vi "T7_WriteRead_FLOAT32_Test_Register.vi"() -> ()   [LabVIEW 2014]
uses:
  Serial Link Layer/NI_Modbus_Cleaned/NI Modbus121Clean.llb/MB Ethernet Master Query Read Input Registers (poly).vi
  Serial Link Layer/NI_Modbus_Cleaned/NI Modbus121Clean.llb/MB Ethernet Master Query Write Multiple Registers (poly).vi
panel:
  in  "LabJack TestFLOAT32 Register":i32=55124
  out "Read FLOAT32":sgl
  out "Raw Data Read":u16[](array[numeric])
  in  "FLOAT32 to Write":sgl=1.23
  in  "WriteData":bool
  in  "Remote IP Address":string="192.168.1.15"
  in  "Remote Port":u16=502
  in  "Stop":bool
  # "MB Ethernet Example Master.vi\n\nInstructions\n1.Use Kipling to find your devices IP address & modify the\n\"Remote IP Addres\"\n2. Run this VI\n3. Change value of \"FLOAT32 to Write\" & press \"Write Data\""
  # "TCP Parameters"
  # "Test Write & Read of TEST_UINT32 Register"
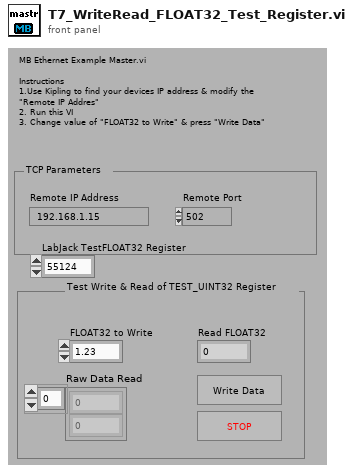
[diagram p1: front panel]
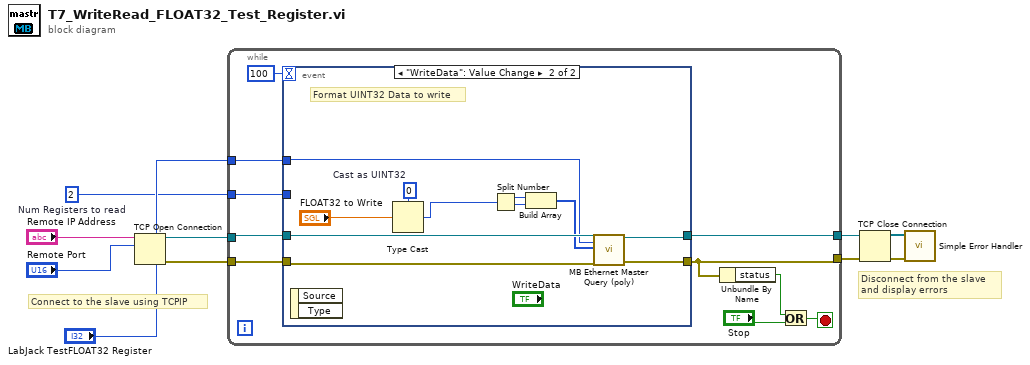
[diagram p0: block diagram]
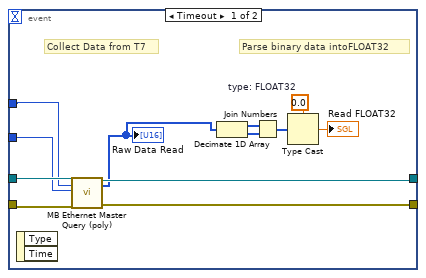
[diagram p2: hidden frame]
diagram:
  w1 = 2  # Num Registers to read
  # "Disconnect from the slave\nand display errors"
  # "Connect to the slave using TCPIP"
  n1 = TCP Open Connection(address="Remote IP Address", remote port or service name="Remote Port") -> (connection ID=w7:refnum<k5>, error out=w6:errorcluster)  [unwired: 3 in]
  n2 = while {
    tunnel: [w16] -> w4
    tunnel: w7 -> [w14]
    tunnel: w6 -> [w13]
    tunnel: [w12] -> w3
    tunnel: "LabJack TestFLOAT32 Register" -> [w11]
    tunnel: w1 -> [w10]
    stop <- w19 stop-if-true
    n3 = event shown="[1] \"WriteData\": Value Change" {
      selector: _ -> [_ _]
      dyn-events: _ -> [_ _]
      timeout: 100 -> [_ _]
      tunnel: [w28 w39] -> w16
      tunnel: w14 -> [w31 w42]
      tunnel: w13 -> [w30 w41]
      tunnel: [w29 w40] -> w12
      tunnel: w11 -> [w27 w38]
      tunnel: w10 -> [w26 _]
      event Timeout {
        w21 = sgl 0.0  # type: FLOAT32
        # "Parse binary data intoFLOAT32"
        # "Collect Data from T7"
        n4 = event-data() -> ()  [unwired: 3 out]
        n5 = call-poly "MB Ethernet Master Query (poly).vi"("TCP Connection Refnum in"=w31, "Starting Address"=w27, "Quantity"=w26, "error in"=w30) -> ("TCP Connection Refnum (dup)"=w29:refnum<k5>, "Input Registers"=w23:u16[], "error out"=w28:errorcluster)  [unwired: 12 in, 1 out]
        "Raw Data Read" <- w23
        n6 = Decimate 1D Array(w23) -> (w25:u16[], w24:u16[])
        n7 = Join Numbers(hi=w25, lo=w24) -> ((hi.lo)=w22:u32[])
        n8 = Type Cast(type=w21, x=w22) -> (*(type *) &x=→"Read FLOAT32":sgl)
      }
      event "WriteData": Value Change {
        w35 = u32 0  # Cast as UINT32
        # "Format UINT32 Data to write"
        n9 = event-data() -> ()  [unwired: 3 out]
        n10 = Type Cast(type=w35, x="FLOAT32 to Write") -> (*(type *) &x=w34:u32)
        n11 = Split Number(x=w34) -> (hi(x)=w33:u16, lo(x)=w32:u16)
        n12 = Build Array(w33, w32) -> (w37:u16[])
        n13 = call-poly "MB Ethernet Master Query (poly).vi"("TCP Connection Refnum in"=w42, "Starting Address"=w38, "Registers"=w37, "error in"=w41) -> ("TCP Connection Refnum (dup)"=w40:refnum<k5>, "error out"=w39:errorcluster)  [unwired: 13 in, 1 out]
      }
    }
    n14 = Unbundle By Name(w16) -> ("status"=w17:bool)
    n15 = Or(x=w17, y="Stop") -> (x .or. y?=w19:bool)
  }
  n16 = TCP Close Connection(connection ID=w3, error in (no error)=w4) -> (error out=w5:errorcluster)  [unwired: 2 out]
  n17 = call <vilib>:"Simple Error Handler.vi"("error in (no error)"=w5) -> ()  [unwired: 1 in, 8 out]
